vi "Color_HighlightComments.vi"(11 "String in":refnum<vi>) -> (3 "String out":refnum<vi>)   [LabVIEW 2022 SP3]
uses:
  Color_Globals.vi
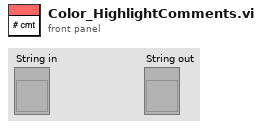
[diagram p1: front panel]
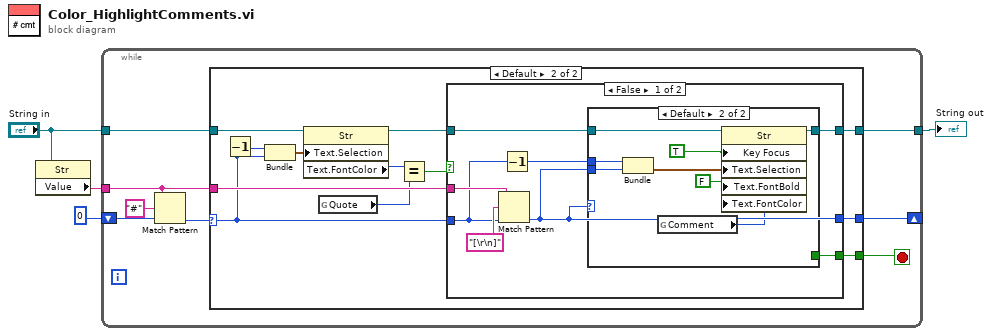
[diagram p0: block diagram]
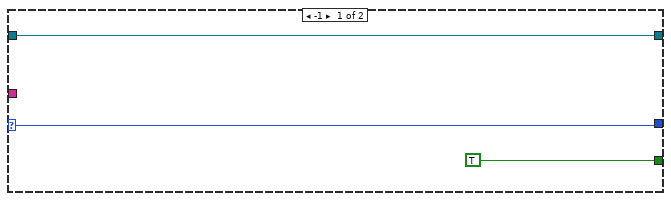
[diagram p2: hidden frame]
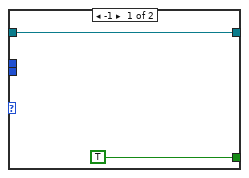
[diagram p3: hidden frame]
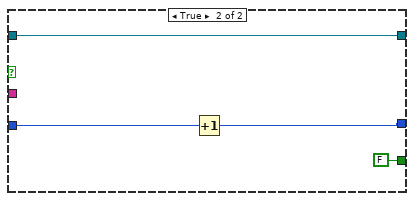
[diagram p4: hidden frame]
diagram:
  n1 = property on="Property Node" class="Str"(reference="String in") -> ("Value"=w1:string)  [unwired: 1 in, 2 out]
  n2 = while {
    tunnel: w1 -> [w9]
    shift-right: [w10] -> _
    shift-left: 0 -> [w12]
    tunnel: "String in" -> [w5]
    tunnel: [w8] -> w4
    stop <- w7 stop-if-true
    n3 = Match Pattern(string=w9, regular expression="#", offset (0)=w12) -> (offset past match=w6:i32)  [unwired: 3 out]
    n4 = case shown="Default" w6 {
      selector: w6 -> [w14 w20]
      tunnel: [w14 w25] -> w10
      tunnel: w5 -> [w15 w19]
      tunnel: w9 -> [_ w27]
      tunnel: [w15 w26] -> w8
      tunnel: [TRUE w24] -> w7
      frame -1 {
      }
      frame Default {
        n5 = Decrement(x=w20) -> (x-1=w23:i32)
        n6 = Bundle(w23, "offset past match"=w20) -> (w22:cluster{i32, "offset past match":i32})  [unwired: 1 in]
        n7 = property on="Property Node" class="Str"(reference=w19, "Text.Selection"=w22) -> (reference out=w18:refnum<vi>, "Text.FontColor"=w21:u32)  [unwired: 1 in, 1 out]
        n8 = global read "Color_Globals.vi" "Quote"() -> (w16:u32)
        n9 = Equal?(x=w21, y=w16) -> (x = y?=w17:bool)
        n10 = case shown="False" w17 {
          tunnel: w27 -> [w33 _]
          tunnel: [w32 w49] -> w26
          tunnel: [w31 w46] -> w25
          tunnel: [w30 FALSE] -> w24
          tunnel: w20 -> [w29 w48]
          tunnel: w18 -> [w28 w49]
          frame False {
            n11 = Match Pattern(string=w33, regular expression="[\r\n]", offset (0)=w29) -> (offset past match=w31:i32)  [unwired: 3 out]
            n12 = Decrement(x=w29) -> (x-1=w34:i32)
            n13 = case shown="Default" w31 {
              tunnel: w31 -> [_ w45]
              tunnel: w28 -> [w36 w39]
              tunnel: w34 -> [_ w41]
              tunnel: [w36 w40] -> w32
              tunnel: [TRUE _] -> w30
              frame -1 {
              }
              frame Default {
                n14 = Bundle(w41, "offset past match"=w45) -> (w42:cluster{i32, "offset past match":i32})  [unwired: 1 in]
                n15 = global read "Color_Globals.vi" "Comment"() -> (w38:u32)
                n16 = property on="Property Node" class="Str"(reference=w39, "Key Focus"=TRUE, "Text.Selection"=w42, "Text.FontBold"=FALSE ("Text.Font:Bold"), "Text.FontColor"=w38) -> (reference out=w40:refnum<vi>)  [unwired: 1 in, 1 out]
              }
            }
          }
          frame True {
            n17 = Increment(x=w48) -> (x+1=w46:i32)
          }
        }
      }
    }
  }
  "String out" <- w4
